vi "ble_discover_characteristics.vi"(6 "Connection Status":T1={"MAC Address"="", "cnx handle"=0, "cnx flags"=0, "Address Type"=125, "Connection Interval (ms)"=125, "Timeout(ms)"=125, "Latency"=0, "bonding handle"=0} {"Address Type" items=["Public", "Random"]}, 8 "error in (no error)":errorcluster, 11 "COM Bluegiga in":refnum<visa-resource-name>) -> (0 "error out":errorcluster, 2 "characteristics_info":u8[][](array[numeric]), 3 "COM Bluegiga out":refnum<visa-resource-name>)   [LabVIEW 2015]
uses:
  type_def/connection_status_bundle.ctl
  type_def/address_type.ctl
panel:
  in  "Last Handle Number (0xFFFF)":u16=65535 format="%04x"
  in  "First Handle Number(0x0001)":u16=1 format="%04x"
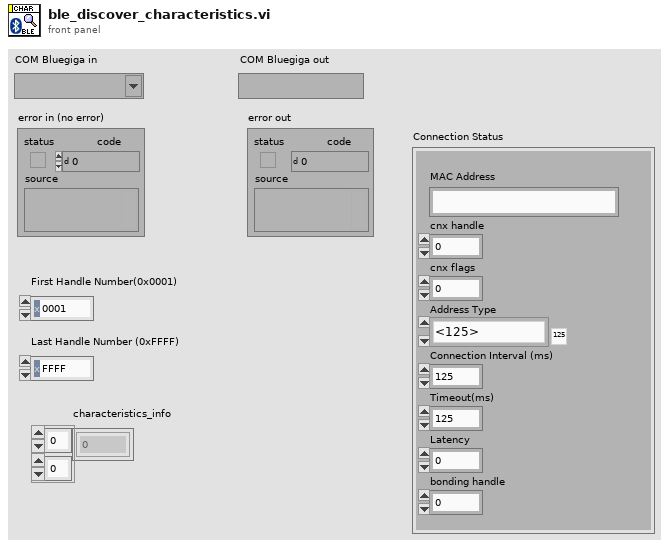
[diagram p1: front panel]
types:
  T1 = typedef "connection_status_bundle.ctl" = cluster{"MAC Address":string, "cnx handle":u8, "cnx flags":u8, "Address Type":T2, "Connection Interval (ms)":u16, "Timeout(ms)":u16, "Latency":u16, "bonding handle":u8}
  T2 = typedef "address_type.ctl" = u8
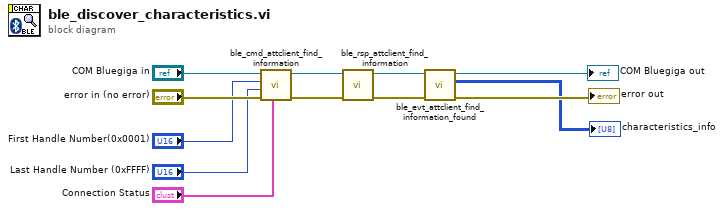
[diagram p0: block diagram]
diagram:
  n1 = call "ble_cmd_attclient_find_information.vi"("Connection Status"="Connection Status", "error in (no error)"="error in (no error)", "Last Handle Number (0xFFFF)"="Last Handle Number (0xFFFF)", "First Handle Number(0x0001)"="First Handle Number(0x0001)", "COM Bluegiga in"="COM Bluegiga in") -> ("error out"=w12:errorcluster, "COM Bluegiga out"=w8:refnum<visa-resource-name>)  [unwired: 5 in]
  n2 = call "ble_rsp_attclient_find_information.vi"("error in (no error)"=w12, "COM Bluegiga in"=w8) -> ("error out"=w11:errorcluster, "COM Bluegiga out"=w7:refnum<visa-resource-name>)  [unwired: 6 in, 2 out]
  n3 = call "ble_evt_attclient_find_information_found.vi"("error in (no error)"=w11, "COM Bluegiga in"=w7) -> ("error out"=→"error out":errorcluster, "characteristics_info"=→"characteristics_info":u8[][], "COM Bluegiga out"=→"COM Bluegiga out":refnum<visa-resource-name>)  [unwired: 7 in]
